vi "create.vi"(5 "Reference":string, 7 "Date":timestamp, 8 "error in (no error)":errorcluster, 9 "Category":string, 10 "Description":string, 11 "Amount":dbl) -> (0 "error out":errorcluster, 3 "Credit Transaction out":refnum<class "CreditTransaction.lvclass">)   [LabVIEW 2018, in "CreditTransaction.lvclass"]
uses:
  CreditTransaction.lvclass
  C:/GitRepos/Filthy-Lucre-Budgetizer/source/support/classes/Transaction/Transaction.lvclass
  Transaction/Transaction.lvclass
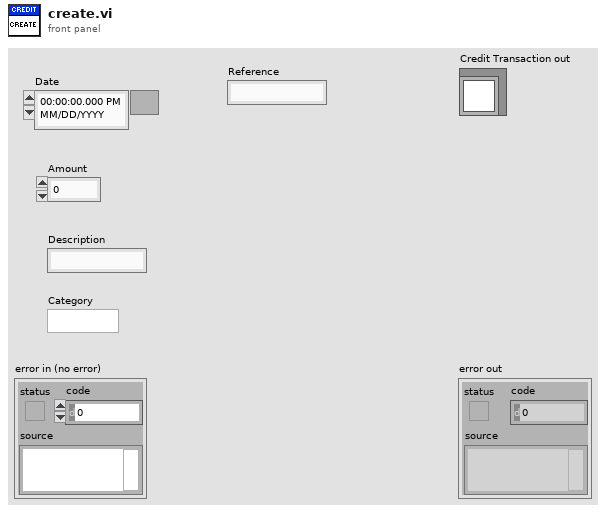
[diagram p1: front panel]
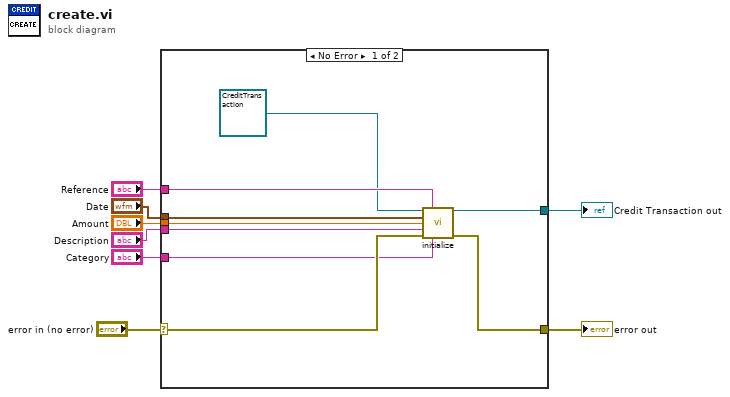
[diagram p0: block diagram]
diagram:
  n1 = case shown="No Error" "error in (no error)" {
    selector: "error in (no error)" -> [w13 w18]
    tunnel: [w12 w18] -> w7
    tunnel: "Reference" -> [w17 _]
    tunnel: "Date" -> [w16 _]
    tunnel: "Amount" -> [w15 _]
    tunnel: "Description" -> [w14 _]
    tunnel: "Category" -> [w11 _]
    tunnel: [w9 _] -> w1
    frame No Error {
      n2 = call "initialize.vi"("Transaction in"=refnum<class "CreditTransaction.lvclass"> refnum ("Credit Transaction in"), "Reference"=w17, "Date"=w16, "Amount"=w15, "Description"=w14, "error in (no error)"=w13, "Category"=w11) -> ("Transaction out"=w9:refnum<class "CreditTransaction.lvclass">, "error out"=w12:errorcluster)  [unwired: 7 in]
    }
    frame Error {
    }
  }
  "error out" <- w7
  "Credit Transaction out" <- w1
